vi "Log Data.vi"(8 "error in (no error)":errorcluster, 9 "Samples to Save In":u32, 10 "Data":waveform(dbl)[](array[waveform]), 11 "Logging Configuration":T1) -> (0 "error out":errorcluster, 1 "Samples to Save Out":u32)   [LabVIEW 2016, in "Logging.lvlib"]
doc: "Use the Write To Measurement File Express VI to log data to disk in a LVM file."
uses:
  Logging.lvlib
  Logging Configuration.ctl
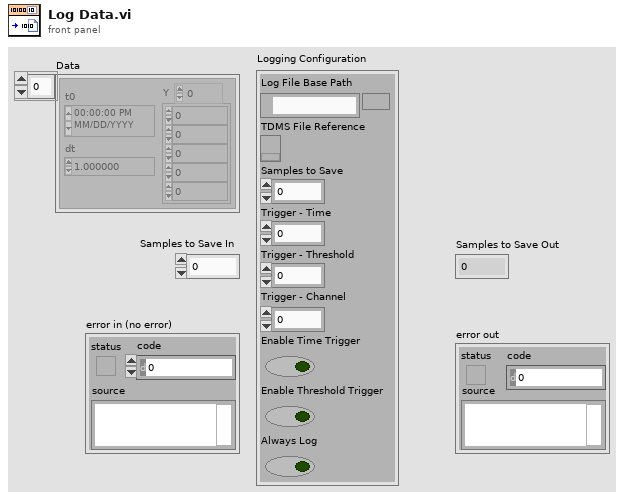
[diagram p1: front panel]
types:
  T1 = typedef "Logging.lvlib/Logging Configuration.ctl" = cluster{"Log File Base Path":path, "TDMS File Reference":refnum<k34>, "Samples to Save":u32, "Trigger - Time":u32, "Trigger - Threshold":dbl, "Trigger - Channel":u32, "Enable Time Trigger":bool, "Enable Threshold Trigger":bool, "Always Log":bool}
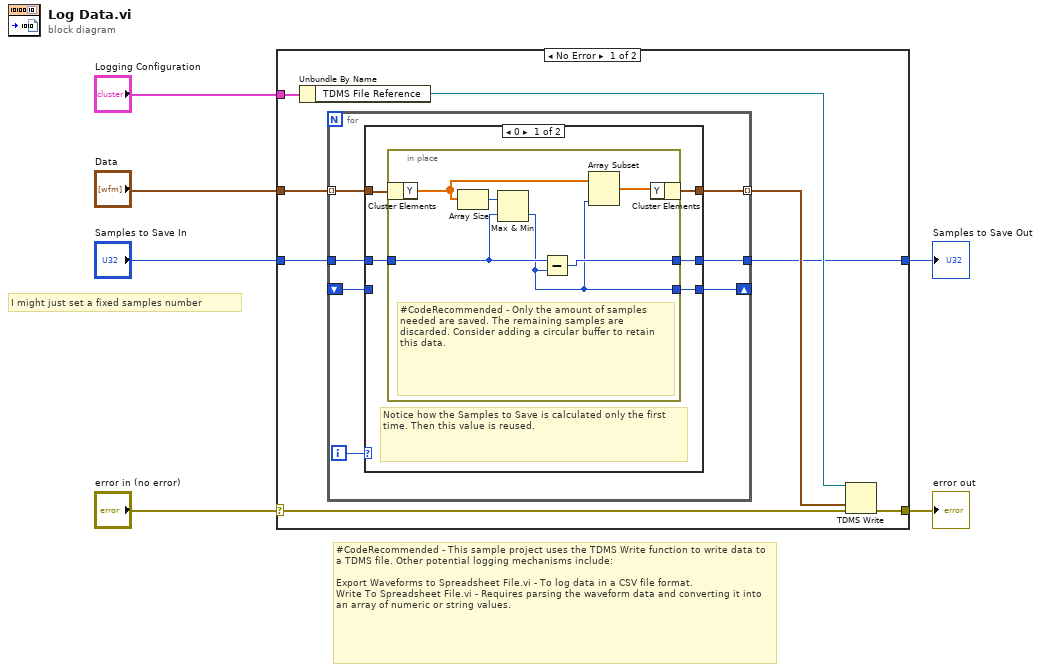
[diagram p0: block diagram]
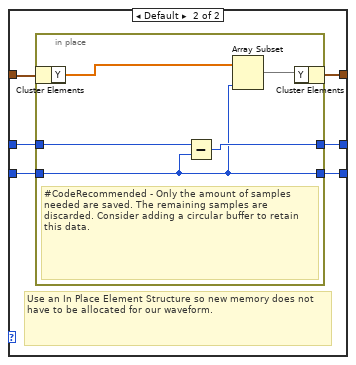
[diagram p2: hidden frame]
diagram:
  # "I might just set a fixed samples number"
  # "#CodeRecommended - This sample project uses the TDMS Write function to write data to a TDMS file. Other potential logging mechanisms include:\n\nExport Waveforms to Spreadsheet File.vi - To log data in a CSV file format.\nWrite To Spreadsheet File.vi - Requires parsing the waveform data and converting it into an array of numeric or string values."
  n1 = case shown="No Error" "error in (no error)" {
    selector: "error in (no error)" -> [w11 w45]
    tunnel: "Logging Configuration" -> [w14 _]
    tunnel: "Data" -> [w10 _]
    tunnel: [w12 w45] -> w5
    tunnel: "Samples to Save In" -> [w9 w44]
    tunnel: [w7 w44] -> w1
    frame No Error {
      n2 = Unbundle By Name(w14) -> ("TDMS File Reference"=w13:refnum<k34>)
      n3 = for {
        tunnel: w10 -> [w20] mode=indexing
        tunnel: w9 -> [w21]
        tunnel: [w19] -> w8 mode=indexing
        tunnel: [w18] -> w7
        shift-right: [w16] -> _
        shift-left: _ -> [w15]
        i -> [w17]
        n4 = case shown="0" w17 {
          tunnel: w21 -> [w26 w38]
          tunnel: w20 -> [w22 w34]
          tunnel: [w23 w33] -> w19
          tunnel: [w25 w37] -> w18
          tunnel: [w24 w35] -> w16
          tunnel: w15 -> [_ w36]
          frame 0 {
            # "Notice how the Samples to Save is calculated only the first time. Then this value is reused."
            n5 = in-place {
              in-place-border: w26 -> [w31]
              in-place-border: [w30] -> w25
              in-place-border: [w27] -> w24
              # "#CodeRecommended - Only the amount of samples needed are saved. The remaining samples are discarded. Consider adding a circular buffer to retain this data."
              n6 = in-place-cluster #1(w22) -> ("Y"=w29:dbl[])
              n7 = Array Size(array=w29) -> (size(s)=w32:i32)
              n8 = Max & Min(x=w32, y=w31) -> (min(x,y)=w27:u32)  [unwired: 1 out]
              n9 = Subtract(x=w31, y=w27) -> (x-y=w30:u32)
              n10 = Array Subset(array=w29, length=w27) -> (w28:dbl[])  [unwired: 1 in]
              n11 = in-place-cluster #1("Y"=w28) -> (w23:waveform(dbl))
            }
          }
          frame Default {
            # "Use an In Place Element Structure so new memory does not have to be allocated for our waveform."
            n12 = in-place {
              in-place-border: w38 -> [w43]
              in-place-border: [w42] -> w37
              in-place-border: [w39] -> w35
              in-place-border: w36 -> [w39]
              # "#CodeRecommended - Only the amount of samples needed are saved. The remaining samples are discarded. Consider adding a circular buffer to retain this data."
              n13 = in-place-cluster #2(w34) -> ("Y"=w41:dbl[])
              n14 = Subtract(x=w43, y=w39) -> (x-y=w42:u32)
              n15 = Array Subset(array=w41, length=w39) -> (w40:dbl[])  [unwired: 1 in]
              n16 = in-place-cluster #2("Y"=w40) -> (w33:waveform(dbl))
            }
          }
        }
      }
      n17 = TDMS Write(0:w13, 9:w8, 11:w11) -> (15:w12:errorcluster)  [unwired: 3 in, 3 out]
    }
    frame Error {
    }
  }
  "error out" <- w5
  "Samples to Save Out" <- w1
